vi "Teleop.vi"(0 "Call Context":T6) -> (9 "SubState 1":T5, 14 "SubState 0":T4=enum."driver control", 16 "Loop 0 Data":T3)   [LabVIEW 2013]
uses:
  typedefs/subStates.ctl
  <vilib>/Rock Robotics/WPI/DriverStation/WPI_DriverStationDerivedRobotMode.ctl
  typedefs/singleUseSubstate.ctl
  typedefs/Loop Datatypes/Loop 0 Datatype.ctl
  <vilib>/Rock Robotics/WPI/Joystick/WPI_JoystickDevRef.ctl
  <vilib>/Rock Robotics/WPI/Joystick/WPI_JoystickDeviceEnum.ctl
  typedefs/fg_typedef.ctl
  typedefs/vision enable.ctl
  <vilib>/Rock Robotics/WPI/Joystick/WPI_JoystickGetSetRefNum.vi
panel:
  out "JS3":T1
  out "JS1":T1
  out "JS2":T1
  out "Exit Value":i32=-1
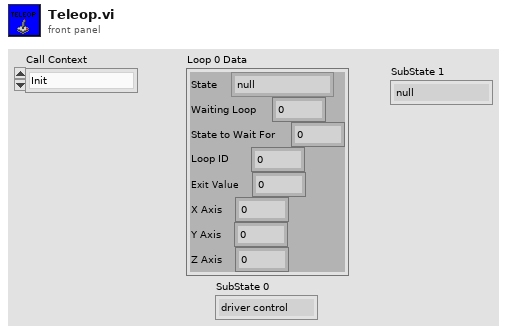
[diagram p1: front panel]
types:
  T1 = typedef "WPI_JoystickDevRef.ctl" = cluster{"Device":T2}
  T2 = typedef "WPI_JoystickDeviceEnum.ctl" = enum16{"USB 1", "USB 2", "USB 3", "USB 4", "Kinect 1", "Kinect 2"}
  T3 = typedef "Loop 0 Datatype.ctl" = cluster{"State":T4, "Waiting Loop":i32, "State to Wait For":i32, "Loop ID":i32, "Exit Value":i32, "X Axis":dbl, "Y Axis":dbl, "Z Axis":dbl}
  T4 = typedef "subStates.ctl" = enum16{"null", "wait", "driver control", "auto", "manual override", "hold position", "rotate", "pickup", "pass", "load", "goto shoot", "shoot", "end"}
  T5 = typedef "singleUseSubstate.ctl" = enum16{"null", "wait", "shift high", "shift low"}
  T6 = typedef "WPI_DriverStationDerivedRobotMode.ctl" = enum16{"Init", "Execute", "Stop"}
  T7 = cluster{"axis 1 (x)":dbl, "axis 2 (y)":dbl, "axis 3 (throttle)":dbl, "axis 4":dbl, "axis 5":dbl, "axis 6":dbl}
  T8 = typedef "vision enable.ctl" = enum16{"Enable", "Disable", "Stop"}
  T9 = typedef "fg_typedef.ctl" = enum16{"Get", "Set"}
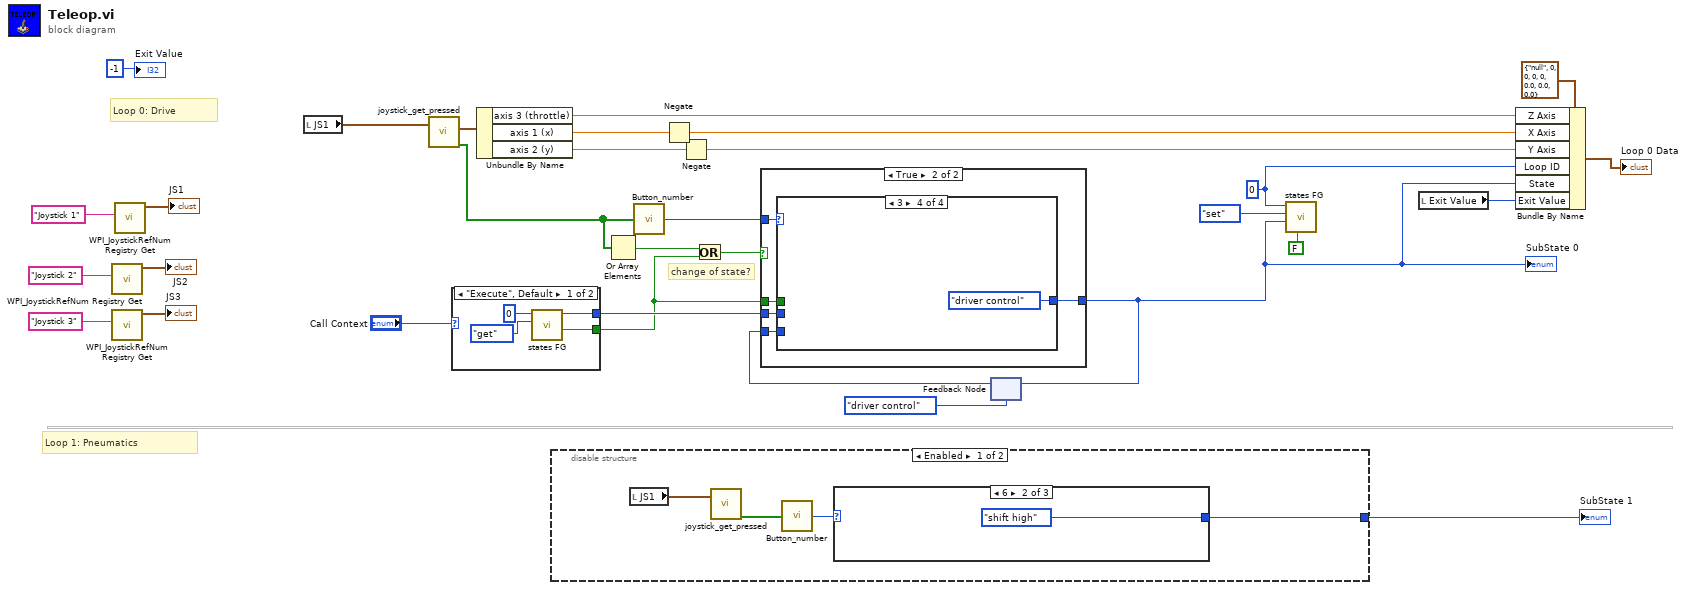
[diagram p0: block diagram]
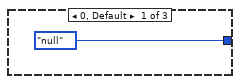
[diagram p2: hidden frame]
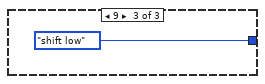
[diagram p3: hidden frame]
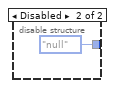
[diagram p4: hidden frame]
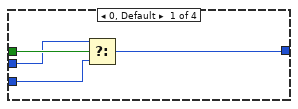
[diagram p6: hidden frame]
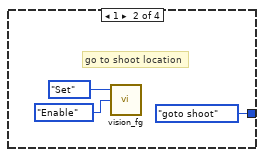
[diagram p7: hidden frame]
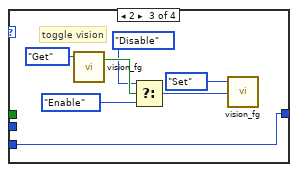
[diagram p8: hidden frame]
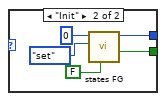
[diagram p9: hidden frame]
diagram:
  w25 = 0 ("Loop ID")
  # "change of state?"
  # "Loop 1: Pneumatics"
  # "Loop 0: Drive"
  n1 = call <vilib>:"WPI_JoystickRefNum Registry Get.vi"("refnum name"="Joystick 2") -> ("JoystickDevRef"=→"JS2":T1)  [unwired: 9 in, 1 out]
  n2 = call <vilib>:"WPI_JoystickRefNum Registry Get.vi"("refnum name"="Joystick 3") -> ("JoystickDevRef"=→"JS3":T1)  [unwired: 9 in, 1 out]
  n3 = call <vilib>:"WPI_JoystickRefNum Registry Get.vi"("refnum name"="Joystick 1") -> ("JoystickDevRef"=→"JS1":T1)  [unwired: 9 in, 1 out]
  n4 = local read "JS1"() -> (w8:T1)
  n5 = call "joystick_get_pressed.vi"("JoystickDevRef 2"=w8) -> ("Axes"=w14:T7, "Buttons Pressed?"=w3:bool[])  [unwired: 1 in, 2 out]
  n6 = case shown="\"Execute\", Default" "Call Context" {
    tunnel: [w33 w38] -> w6
    tunnel: [w32 w36] -> w27
    frame "Execute", Default {
      n7 = call "states FG.vi"("menu (get)"=enum16{"set", "get"}."get", "Loop ID"=0) -> ("exit out"=w33:bool, "subState out"=w32:T4)  [unwired: 6 in, 2 out]
    }
    frame "Init" {
      n8 = call "states FG.vi"("exit in"=FALSE, "menu (get)"=enum16{"set", "get"}."set", "Loop ID"=0) -> ("exit out"=w38:bool, "subState out"=w36:T4)  [unwired: 5 in, 2 out]
    }
  }
  n9 = Unbundle By Name(w14) -> ("axis 3 (throttle)"=w4:dbl, "axis 1 (x)"=w18:dbl, "axis 2 (y)"=w17:dbl)
  n10 = disable-structure shown="Enabled" {
    disable-tunnel: [w42 singleUseSubstate."null" ("SubState 5")] -> w21
    frame Enabled {
      n11 = local read "JS1"() -> (w41:T1)
      n12 = call "joystick_get_pressed.vi"("JoystickDevRef 2"=w41) -> ("Buttons Pressed?"=w44:bool[])  [unwired: 1 in, 3 out]
      n13 = call "Button_number.vi"("Button Array"=w44) -> ("Button Pressed"=w43:i32)
      n14 = case shown="6" w43 {
        tunnel: [singleUseSubstate."null" ("Enum") singleUseSubstate."shift high" ("Enum") singleUseSubstate."shift low" ("Enum")] -> w42
        frame 0, Default {
        }
        frame 6 {
        }
        frame 9 {
        }
      }
    }
    frame Disabled {
    }
  }
  "SubState 1" <- w21
  n15 = Or Array Elements(Boolean array=w3) -> (logical OR=w7:bool)
  n16 = call "Button_number.vi"("Button Array"=w3) -> ("Button Pressed"=w13:i32)
  n17 = Negate(x=w18) -> (-x=w16:dbl)
  n18 = Negate(x=w17) -> (-x=w15:dbl)
  n19 = Or(x=w7, y=w6) -> (x .or. y?=w5:bool)
  n20 = feedback #1(subStates."driver control" ("Drive SubState")) -> (w28:T4)
  n21 = case shown="True" w5 {
    tunnel: w28 -> [w49 w51]
    tunnel: [w49 w50] -> w1
    tunnel: w27 -> [_ w52]
    tunnel: w13 -> [_ w54]
    tunnel: w6 -> [_ w53]
    frame False {
      # "keep current state, no change necessary"
    }
    frame True {
      n22 = case shown="3" w54 {
        tunnel: w53 -> [w58 _ _ _]
        tunnel: w52 -> [w57 _ _ _]
        tunnel: w51 -> [w56 _ w68 _]
        tunnel: [w55 subStates."goto shoot" ("Drive SubState") w68 subStates."driver control" ("Drive SubState")] -> w50
        frame 0, Default {
          n23 = Select(t=w57, s=w58, f=w56) -> (s? t:f=w55:T4)
        }
        frame 1 {
          # "go to shoot location"
          n24 = call "vision_fg.vi"("Action"=vision_enable."Enable", "Menu"=fg_typedef."Set") -> ()  [unwired: 1 in, 2 out]
        }
        frame 2 {
          # "toggle vision"
          n25 = call "vision_fg.vi"("Menu"=fg_typedef."Get") -> ("Enabled?"=w66:bool)  [unwired: 2 in, 1 out]
          n26 = Select(t=vision_enable."Disable" ("Action"), s=w66, f=vision_enable."Enable" ("Action")) -> (s? t:f=w62:T8)
          n27 = call "vision_fg.vi"("Action"=w62, "Menu"=fg_typedef."Set") -> ()  [unwired: 1 in, 2 out]
        }
        frame 3 {
        }
      }
    }
  }
  "SubState 0" <- w1
  n28 = feedback-in #1(w1) -> ()
  n29 = call "states FG.vi"("exit in"=FALSE, "subState in"=w1, "menu (get)"=enum16{"set", "get"}."set", "Loop ID"=w25) -> ()  [unwired: 4 in, 4 out]
  n30 = local read "Exit Value"() -> (w23:i32)
  n31 = Bundle By Name(cluster=T3 {"State"=enum."null", "Waiting Loop"=0, "State to Wait For"=0, "Loop ID"=0, "Exit Value"=0, "X Axis"=0.0, "Y Axis"=0.0, "Z Axis"=0.0} ("Cluster"), "Z Axis"=w4, "X Axis"=w16, "Y Axis"=w15, "Loop ID"=w25, "State"=w1, "Exit Value"=w23) -> (→"Loop 0 Data":T3)
  "Exit Value" <- -1 ("Exit Value")
